vi "serial_exercise.vi"() -> ()   [LabVIEW 2019]
uses:
  <vilib>/Instr/_visa.llb/VISA Configure Serial Port (Instr).vi
  usbtc08.dll
panel:
  in  "?":bool
  in  "Ch # 8":bool
  in  "Type # 8":i16(ring)=107 items=["B"=98, "E"=101, "J"=106, "K"=107, "N"=110, "R"=114, "S"=115, "T"=116, "Voltage"=120]
  in  "Ch # 7":bool
  in  "Type # 7":i16(ring)=107 items=["B"=98, "E"=101, "J"=106, "K"=107, "N"=110, "R"=114, "S"=115, "T"=116, "Voltage"=120]
  in  "Ch # 6":bool
  in  "Type # 6":i16(ring)=107 items=["B"=98, "E"=101, "J"=106, "K"=107, "N"=110, "R"=114, "S"=115, "T"=116, "Voltage"=120]
  in  "Ch # 5":bool
  in  "Type # 5":i16(ring)=107 items=["B"=98, "E"=101, "J"=106, "K"=107, "N"=110, "R"=114, "S"=115, "T"=116, "Voltage"=120]
  in  "Ch # 4":bool
  in  "Type # 4":i16(ring)=107 items=["B"=98, "E"=101, "J"=106, "K"=107, "N"=110, "R"=114, "S"=115, "T"=116, "Voltage"=120]
  in  "Ch # 3":bool
  in  "Type # 3":i16(ring)=107 items=["B"=98, "E"=101, "J"=106, "K"=107, "N"=110, "R"=114, "S"=115, "T"=116, "Voltage"=120]
  in  "Ch# 2":bool=TRUE
  in  "Type # 2":i16(ring)=107 items=["B"=98, "E"=101, "J"=106, "K"=107, "N"=110, "R"=114, "S"=115, "T"=116, "Voltage"=120]
  in  "Ch# 1":bool=TRUE
  in  "Type # 1":i16(ring)=107 items=["B"=98, "E"=101, "J"=106, "K"=107, "N"=110, "R"=114, "S"=115, "T"=116, "Voltage"=120]
  in  "Units":enum16{"C°", "F°", "K°", "R°"}(ring)
  in  "stop":bool
  out "?":dynamicdata(graph)
  out "Min Interval (ms)":i32
  out "Handle":i16
  in  "Mains Frequency":i16(ring) items=["50 Hz", "60 Hz"]
  in  "Quit":bool
  out "Received Messages:":string
  in  "Sent":bool
  in  "Type new message here:":string
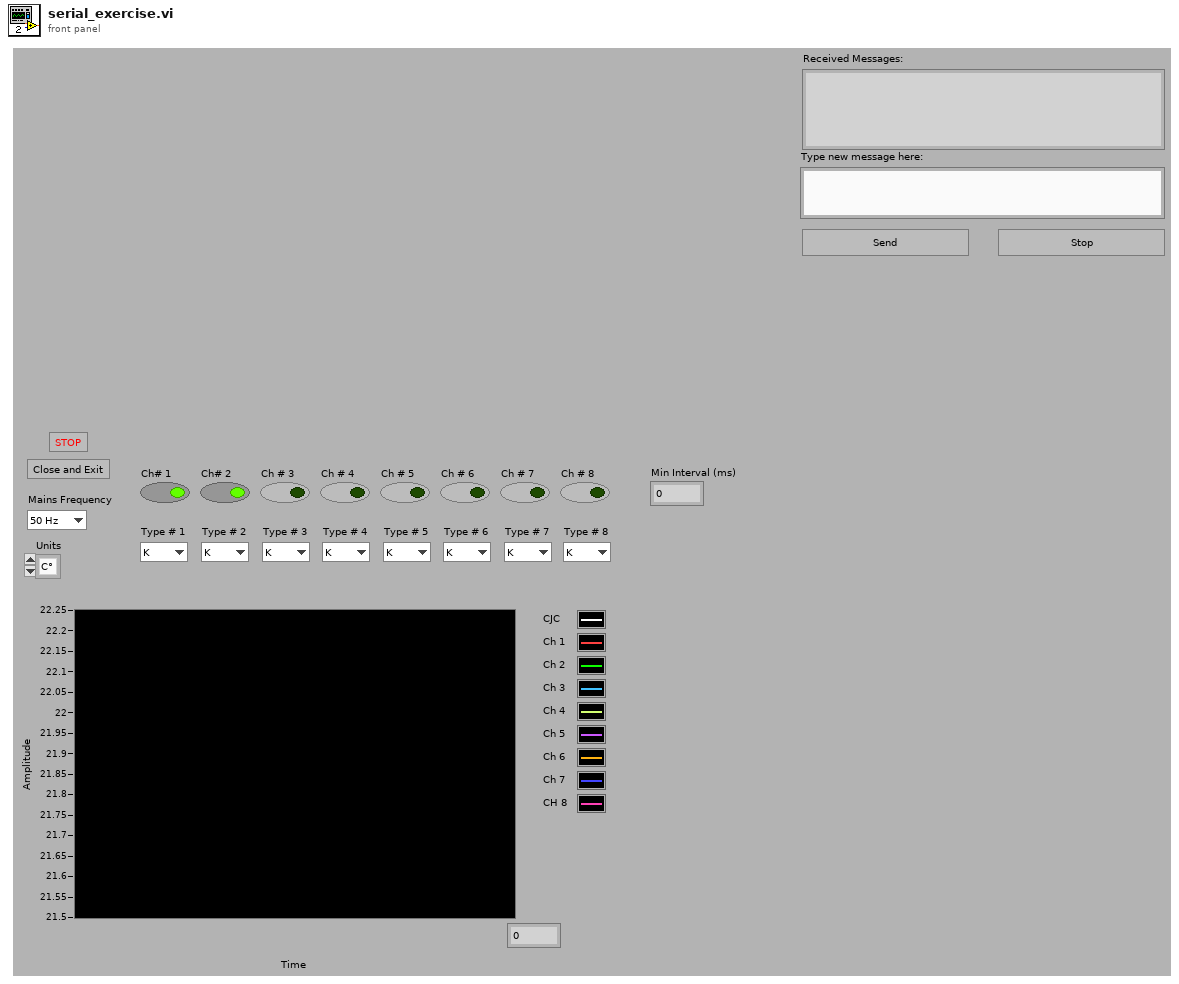
[diagram p1: front panel]
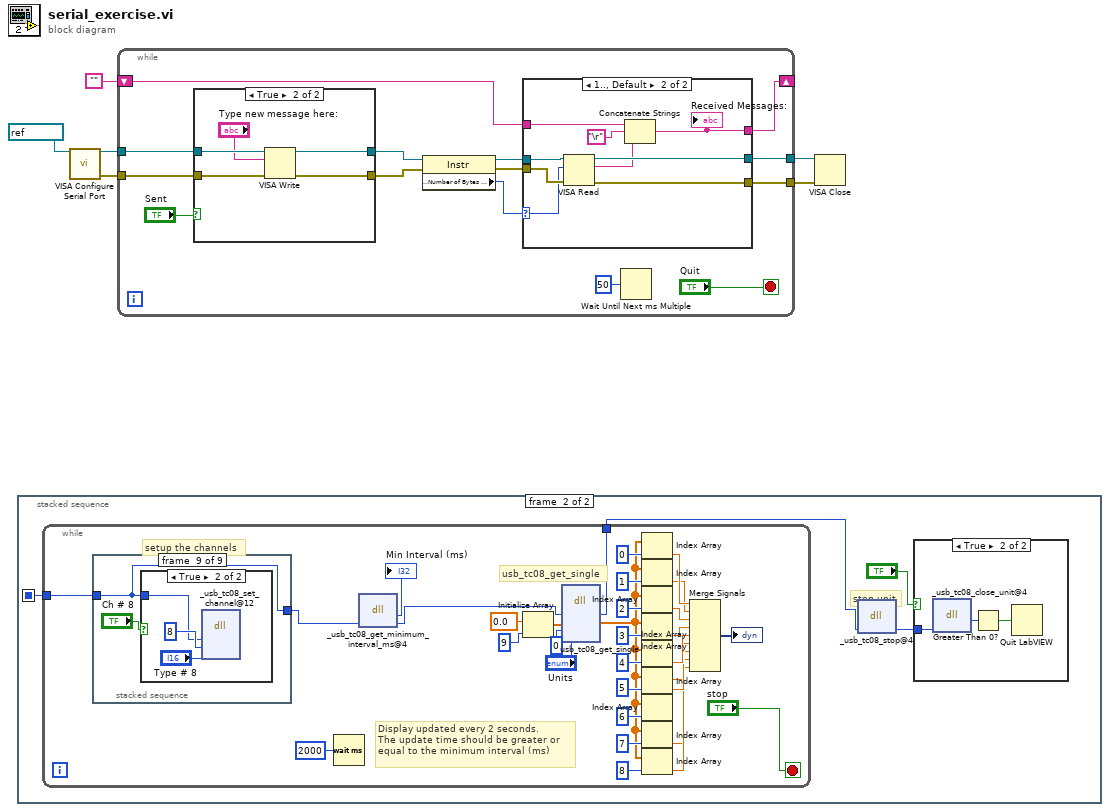
[diagram p0: block diagram]
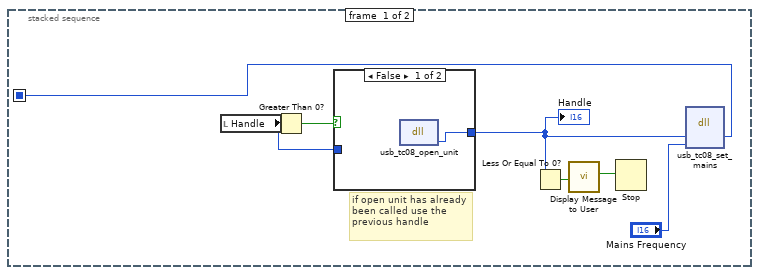
[diagram p2: hidden frame]
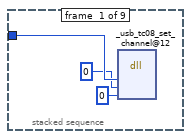
[diagram p4: hidden frame]
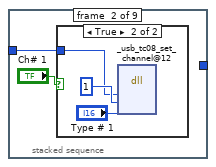
[diagram p5: hidden frame]
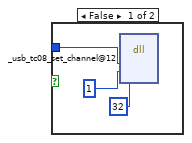
[diagram p6: hidden frame]
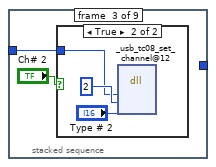
[diagram p7: hidden frame]
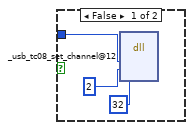
[diagram p8: hidden frame]
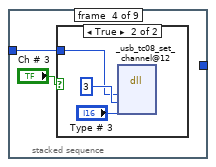
[diagram p9: hidden frame]
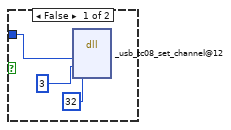
[diagram p10: hidden frame]
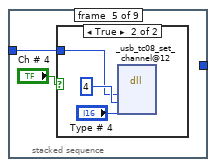
[diagram p11: hidden frame]
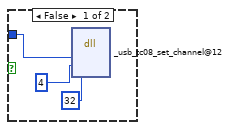
[diagram p12: hidden frame]
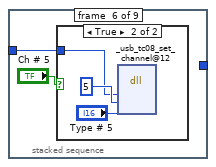
[diagram p13: hidden frame]
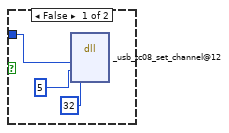
[diagram p14: hidden frame]
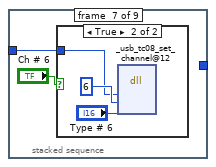
[diagram p15: hidden frame]
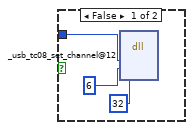
[diagram p16: hidden frame]
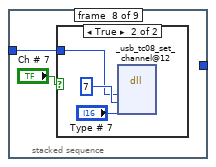
[diagram p17: hidden frame]
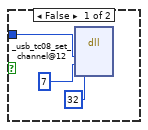
[diagram p18: hidden frame]
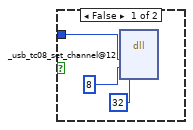
[diagram p19: hidden frame]
diagram:
  n1 = stacked-sequence {
    seq-local: [w11 _] -> [_ w19]
    frame #0 {
      # "if open unit has already been called use the previous handle"
      n2 = local read "Handle"() -> (w12:i16)
      n3 = Greater Than 0?(x=w12) -> (x > 0?=w13:bool)
      n4 = case shown="False" w13 {
        tunnel: [w14 w15] -> w10
        tunnel: w12 -> [_ w15]
        frame False {
          n5 = dll-call lib="usbtc08.dll" fn="usb_tc08_open_unit" label="OpenUnit"() -> ("Handle"=w14:i16)  [unwired: 3 in, 2 out]
        }
        frame True {
        }
      }
      "Handle" <- w10
      n6 = Less Or Equal To 0?(x=w10) -> (x <= 0?=w9:bool)
      n7 = call "Display Message to User"("Enable"=w9) -> ("OK"=w8:bool)  [unwired: 9 in, 1 out]
      n8 = Stop(stop? (T)=w8) -> ()
      n9 = dll-call lib="usbtc08.dll" fn="usb_tc08_set_mains" label="Set Mains"("Handle"=w10, "sixtyHertz"="Mains Frequency") -> ("Handle"=w11:i16)  [unwired: 5 in, 2 out]
    }
    frame #1 {
      # "stop unit"
      n10 = while {
        tunnel: w19 -> [w51]
        tunnel: [w26] -> w16
        stop <- "stop" stop-if-true
        # "Display updated every 2 seconds.\nThe update time should be greater or\nequal to the minimum interval (ms)"
        # "usb_tc08_get_single"
        # "setup the channels"
        n11 = stacked-sequence {
          tunnel: w51 -> [w54 w56 w64 w72 w80 w88 w96 w104 w111]
          tunnel: [_ _ _ _ _ _ _ _ w111] -> w22
          frame #0 {
            n12 = dll-call lib="usbtc08.dll" fn="_usb_tc08_set_channel@12"("handle"=w54, "channel"=i16 0, "tc_type"=i8 0) -> ()  [unwired: 7 in, 2 out]
          }
          frame #1 {
            n13 = case shown="True" "Ch# 1" {
              tunnel: w56 -> [w58 w61]
              frame False {
                n14 = dll-call lib="usbtc08.dll" fn="_usb_tc08_set_channel@12"("handle"=w58, "channel"=i16 1, "tc_type"=32) -> ()  [unwired: 7 in, 2 out]
              }
              frame True {
                n15 = dll-call lib="usbtc08.dll" fn="_usb_tc08_set_channel@12"("handle"=w61, "channel"=i16 1, "tc_type"="Type # 1") -> ()  [unwired: 7 in, 2 out]
              }
            }
          }
          frame #2 {
            n16 = case shown="True" "Ch# 2" {
              tunnel: w64 -> [w65 w69]
              frame False {
                n17 = dll-call lib="usbtc08.dll" fn="_usb_tc08_set_channel@12"("handle"=w65, "channel"=i16 2, "tc_type"=32) -> ()  [unwired: 7 in, 2 out]
              }
              frame True {
                n18 = dll-call lib="usbtc08.dll" fn="_usb_tc08_set_channel@12"("handle"=w69, "channel"=i16 2, "tc_type"="Type # 2") -> ()  [unwired: 7 in, 2 out]
              }
            }
          }
          frame #3 {
            n19 = case shown="True" "Ch # 3" {
              tunnel: w72 -> [w73 w77]
              frame False {
                n20 = dll-call lib="usbtc08.dll" fn="_usb_tc08_set_channel@12"("handle"=w73, "channel"=i16 3, "tc_type"=32) -> ()  [unwired: 7 in, 2 out]
              }
              frame True {
                n21 = dll-call lib="usbtc08.dll" fn="_usb_tc08_set_channel@12"("handle"=w77, "channel"=i16 3, "tc_type"="Type # 3") -> ()  [unwired: 7 in, 2 out]
              }
            }
          }
          frame #4 {
            n22 = case shown="True" "Ch # 4" {
              tunnel: w80 -> [w81 w85]
              frame False {
                n23 = dll-call lib="usbtc08.dll" fn="_usb_tc08_set_channel@12"("handle"=w81, "channel"=i16 4, "tc_type"=32) -> ()  [unwired: 7 in, 2 out]
              }
              frame True {
                n24 = dll-call lib="usbtc08.dll" fn="_usb_tc08_set_channel@12"("handle"=w85, "channel"=i16 4, "tc_type"="Type # 4") -> ()  [unwired: 7 in, 2 out]
              }
            }
          }
          frame #5 {
            n25 = case shown="True" "Ch # 5" {
              tunnel: w88 -> [w89 w93]
              frame False {
                n26 = dll-call lib="usbtc08.dll" fn="_usb_tc08_set_channel@12"("handle"=w89, "channel"=i16 5, "tc_type"=32) -> ()  [unwired: 7 in, 2 out]
              }
              frame True {
                n27 = dll-call lib="usbtc08.dll" fn="_usb_tc08_set_channel@12"("handle"=w93, "channel"=i16 5, "tc_type"="Type # 5") -> ()  [unwired: 7 in, 2 out]
              }
            }
          }
          frame #6 {
            n28 = case shown="True" "Ch # 6" {
              tunnel: w96 -> [w97 w101]
              frame False {
                n29 = dll-call lib="usbtc08.dll" fn="_usb_tc08_set_channel@12"("handle"=w97, "channel"=i16 6, "tc_type"=32) -> ()  [unwired: 7 in, 2 out]
              }
              frame True {
                n30 = dll-call lib="usbtc08.dll" fn="_usb_tc08_set_channel@12"("handle"=w101, "channel"=i16 6, "tc_type"="Type # 6") -> ()  [unwired: 7 in, 2 out]
              }
            }
          }
          frame #7 {
            n31 = case shown="True" "Ch # 7" {
              tunnel: w104 -> [w105 w109]
              frame False {
                n32 = dll-call lib="usbtc08.dll" fn="_usb_tc08_set_channel@12"("handle"=w105, "channel"=i16 7, "tc_type"=32) -> ()  [unwired: 7 in, 2 out]
              }
              frame True {
                n33 = dll-call lib="usbtc08.dll" fn="_usb_tc08_set_channel@12"("handle"=w109, "channel"=i16 7, "tc_type"="Type # 7") -> ()  [unwired: 7 in, 2 out]
              }
            }
          }
          frame #8 {
            n34 = case shown="True" "Ch # 8" {
              tunnel: w111 -> [w113 w117]
              frame False {
                n35 = dll-call lib="usbtc08.dll" fn="_usb_tc08_set_channel@12"("handle"=w113, "channel"=i16 8, "tc_type"=32) -> ()  [unwired: 7 in, 2 out]
              }
              frame True {
                n36 = dll-call lib="usbtc08.dll" fn="_usb_tc08_set_channel@12"("handle"=w117, "channel"=i16 8, "tc_type"="Type # 8") -> ()  [unwired: 7 in, 2 out]
              }
            }
          }
        }
        n37 = Wait (ms)(milliseconds to wait=u32 2000) -> ()  [unwired: 1 out]
        n38 = dll-call lib="usbtc08.dll" fn="_usb_tc08_get_minimum_interval_ms@4"("handle"=w22) -> ("Min Interval (ms)"=→"Min Interval (ms)":i32, "handle"=w21:i16)  [unwired: 3 in, 2 out]
        n39 = Initialize Array(sgl 0.0, i16 9) -> (w50:sgl[])
        n40 = dll-call lib="usbtc08.dll" fn="usb_tc08_get_single"("handle"=w21, "temp_buffer"=w50, "overflow"=i16 0, "units"="Units") -> ("handle"=w26:i16, "temp_buffer"=w36:sgl[])  [unwired: 6 in, 2 out]
        n41 = Index Array(array=w36, index=i16 0) -> (element=w35:sgl)
        n42 = Index Array(array=w36, index=i16 1) -> (element=w25:sgl)
        n43 = Index Array(array=w36, index=i16 2) -> (element=w34:sgl)
        n44 = Index Array(array=w36, index=i16 3) -> (element=w33:sgl)
        n45 = Index Array(array=w36, index=4) -> (element=w32:sgl)
        n46 = Index Array(array=w36, index=i16 5) -> (element=w31:sgl)
        n47 = Index Array(array=w36, index=6) -> (element=w30:sgl)
        n48 = Index Array(array=w36, index=i16 7) -> (element=w28:sgl)
        n49 = Index Array(array=w36, index=i16 8) -> (element=w29:sgl)
        n50 = Merge Signals(w35, w25, w34, w33, w32, w31, w30, w28, w29) -> (→"?":dynamicdata)
      }
      n51 = dll-call lib="usbtc08.dll" fn="_usb_tc08_stop@4" ("Close unit")("handle"=w16) -> ("handle"=w18:i16)  [unwired: 4 in, 2 out]
      n52 = case shown="True" "?" {
        tunnel: w18 -> [_ w121]
        frame False {
        }
        frame True {
          n53 = dll-call lib="usbtc08.dll" fn="_usb_tc08_close_unit@4" ("Close unit")("handle"=w121) -> ("return type"=w120:i16)  [unwired: 4 in, 2 out]
          n54 = Greater Than 0?(x=w120) -> (x > 0?=w119:bool)
          n55 = Quit LabVIEW(quit? (T)=w119) -> ()
        }
      }
    }
  }
  n56 = call-poly "VISA Configure Serial Port"("VISA resource name"=refnum<visa-resource-name> "COM1") -> ("VISA resource name out"=w3:refnum<visa-resource-name>, "error out"=w2:errorcluster)  [unwired: 13 in]
  n57 = while {
    tunnel: w2 -> [w134]
    tunnel: w3 -> [w135]
    shift-left: "" -> [w123]
    shift-right: [w122] -> _
    tunnel: [w125] -> w5
    tunnel: [w124] -> w6
    stop <- "Quit" stop-if-true
    n58 = case shown="True" "Sent" {
      tunnel: w135 -> [w149 w154]
      tunnel: w134 -> [w148 w153]
      tunnel: [w149 w151] -> w130
      tunnel: [w148 w150] -> w129
      frame False {
      }
      frame True {
        n59 = VISA Write(VISA resource name=w154, write buffer="Type new message here:", error in (no error)=w153) -> (VISA resource name out=w151:refnum<visa-resource-name>, error out=w150:errorcluster)  [unwired: 1 out]
      }
    }
    n60 = property class="Instr"(reference=w130, error in=w129) -> (reference out=w126:refnum<visa-resource-name>, error out=w127:errorcluster, "Serial Settings:Number of Bytes at Serial Port"=w128:u32)
    n61 = case shown="1.., Default" w128 {
      selector: w128 -> [_ w145]
      tunnel: w127 -> [w137 w147]
      tunnel: w126 -> [w138 w146]
      tunnel: [w137 w144] -> w125
      tunnel: [w138 w143] -> w124
      tunnel: w123 -> [w136 w140]
      tunnel: [w136 w139] -> w122
      frame 0 {
      }
      frame 1.., Default {
        n62 = VISA Read(VISA resource name=w146, byte count=w145, error in (no error)=w147) -> (VISA resource name out=w143:refnum<visa-resource-name>, read buffer=w141:string, error out=w144:errorcluster)  [unwired: 1 out]
        n63 = Concatenate Strings(w140, "\r", w141) -> (w139:string)
        "Received Messages:" <- w139
      }
    }
    n64 = Wait Until Next ms Multiple(millisecond multiple=u32 50) -> ()  [unwired: 1 out]
  }
  n65 = VISA Close(VISA resource name=w6, error in (no error)=w5) -> ()  [unwired: 1 out]
